vi "例4.10-2 累加（for循环）.vi"() -> ()   [LabVIEW 2017]
panel:
  out "数值":i32
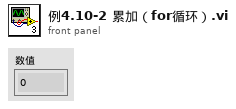
[diagram p1: front panel]
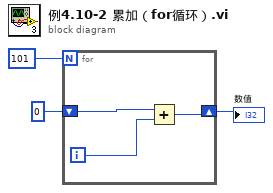
[diagram p0: block diagram]
diagram:
  n1 = for {
    N: 101 -> [_]
    shift-right: [w5] -> w1
    shift-left: 0 -> [w6]
    i -> [w4]
    n2 = Add(x=w6, y=w4) -> (x+y=w5:i32)
  }
  "数值" <- w1
